vi "子VI-查看某框-只读穿透图模式.vi"(0 "输入框号（默认值0为整张图）":dbl format="%#_13g", 1 "框组":T3(array[cluster]), 2 "临界Z值":i32, 4 "临界面积百分比值":dbl, 5 "预先配置的灰度阈值":dbl, 6 "穿透图原始路径":path, 7 "部位信息":string[](array[string])=["", "34.500000", "32.500000", "1121", "34", "54.955926", "分层类", "不合格", ""], 12 "产品规格":cluster{"产品长度（周长）（mm）":dbl, "产品宽度（母线长）（mm）":dbl}) -> (14 "弥散类检测结果":string[][](table), 19 "分层类检测结果":string[][](table))   [LabVIEW 2021]
uses:
  <vilib>/vision/NI_Vision_Development_Module.lvlib
panel:
  in  "返回主界面":bool caption="辅助定性分析"
  out "Pixel Measurements":i32[](array[ring])=[0, 1, 2, 23, 24, 0, 1, 48] items=["Bounding Rect Width", "Bounding Rect Height", "Area"]
  in  "Tab Control":T1
  out "?":T2(plugin-control)
  out "Threshold Image":T2(plugin-control)
  out "Threshold Image":T2(plugin-control)
  in  "格式字符串 3":string="%f"
  in  "分隔符（'\\'代码显示） 2":string="\t"
  out "弥散和分层临界灰度值":i64
  out "弥散缺陷个数":i32
  out "分层缺陷个数":i32
  out "合格？ 弥散类":string="fencengThreshold"
  out "合格？分层类":string="fencengThreshold"
  out "弥散测量结果":dbl[][](array[numeric]) format="%.2f"
  out "?":string
  out "面积 (pixels)":i32
  in  "格式字符串 2":string="%f"
  in  "分隔符（'\\'代码显示）":string="\t"
  out "分层测量结果":dbl[][](array[numeric]) format="%.2f"
  out "缺陷初步分类的临界值":sgl format="%#.3f"
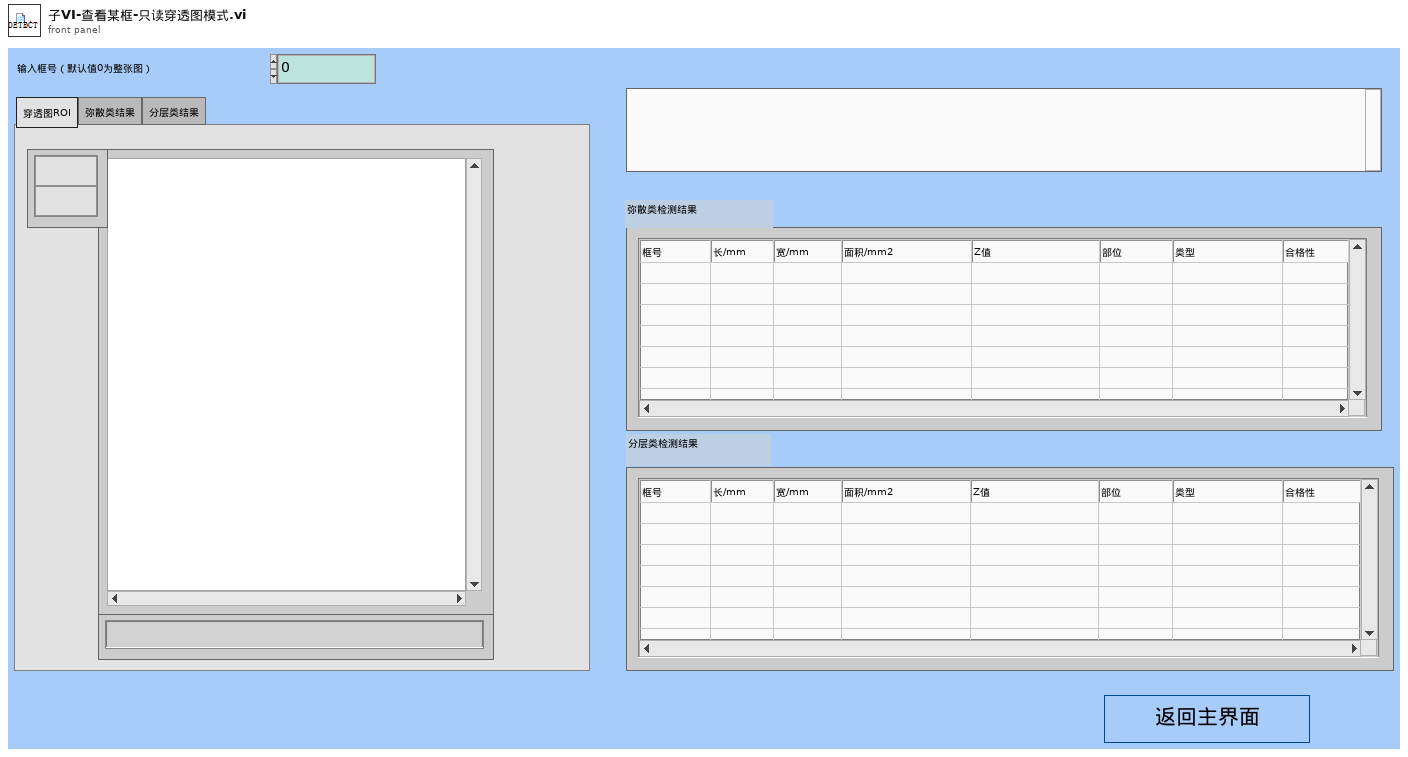
[diagram p1: front panel]
types:
  T1 = typedef "控件2.ctl" = enum32{"穿透图ROI", "弥散类结果", "分层类结果"}
  T2 = typedef "IMAQ Image.ctl" = refnum<image>
  T3 = cluster{"Global Rectangle":i32[], "Contours":cluster{"Contour Type":u32, "ROI Type":u32, "Points":i32[]}[]}[]
  T4 = cluster{"Zoom Tool":bool, "Selection Tool":bool, "Pan Tool":bool, "Point Tool":bool, "Line Tool":bool, "Rectangle Tool":bool, "Rotated Rectangle Tool":bool, "Polyline Tool":bool, "Polygon Tool":bool, "Freehand Tool":bool, "Closed Freehand Tool":bool, "Ellipse Tool":bool, "Annulus Tool":bool}
  T5 = typedef "Image Type" = u32
  T6 = cluster{"Global Rectangle":i32[], "Contours":cluster{"Contour Type":u32, "ROI Type":u32, "Points":i32[]}[]}
  T7 = typedef "Particle Parameters" = i32
  T8 = cluster{"Measurement Parameter":T7, "Range Lower Value":dbl, "Range Upper Value":dbl, "Range":bool, "Measurement Type":bool}[]
  T9 = cluster{"histogram":u32[], "Minimal Value":sgl, "Maximal Value":sgl, "Starting Value":sgl, "Interval Width":sgl, "Mean Value":sgl, "Standard  Variation":sgl, "Area (pixels)":i32}
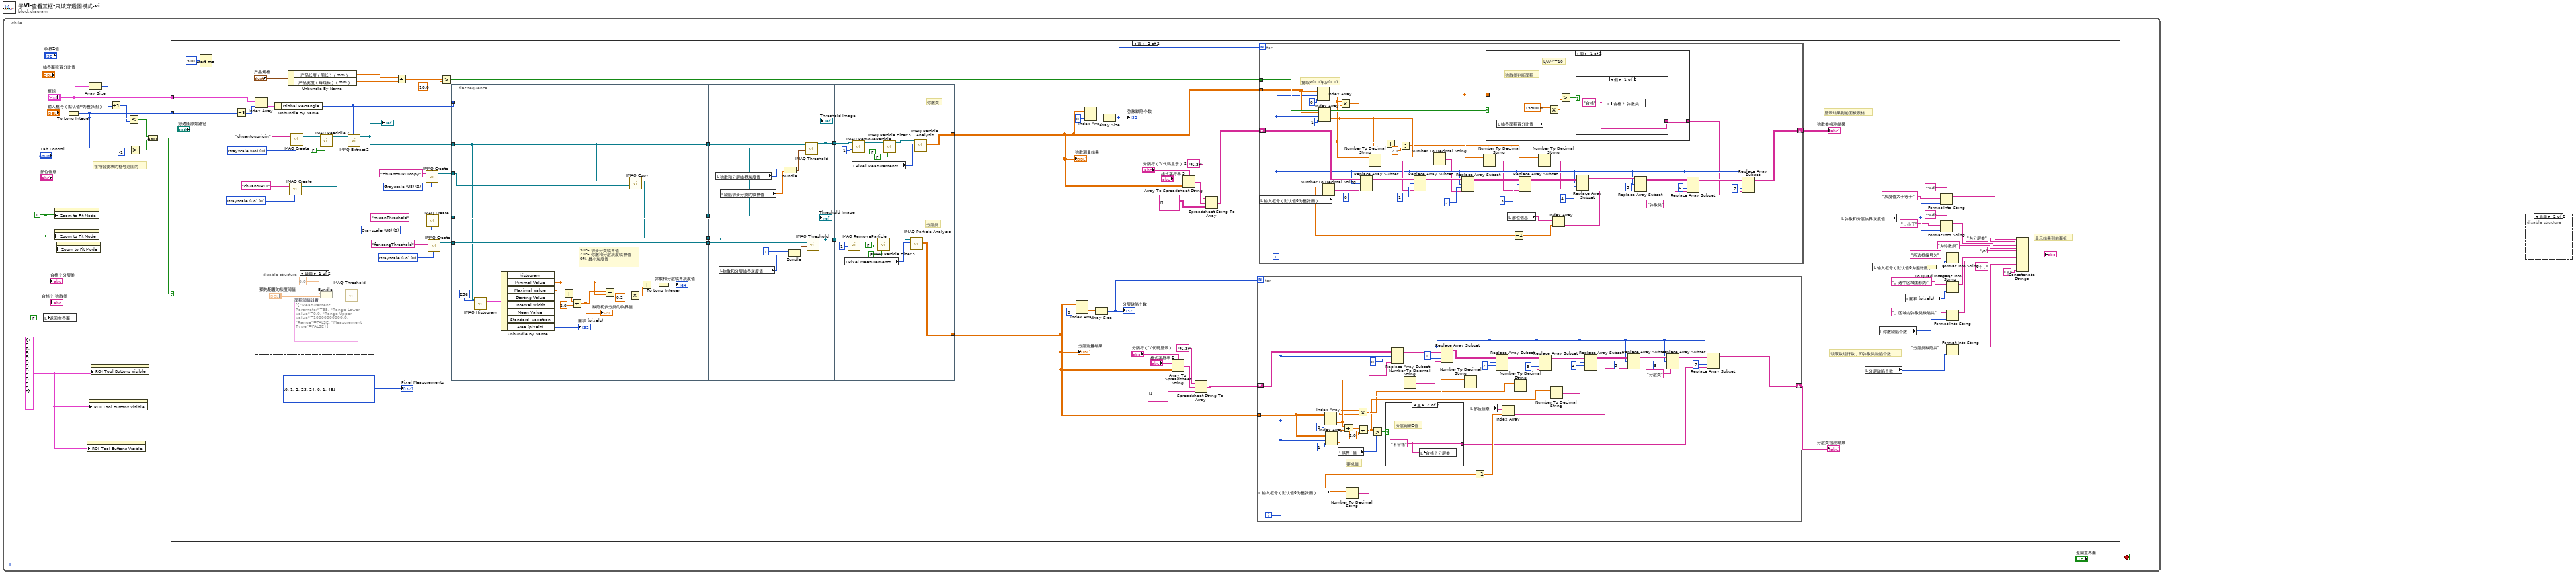
[diagram p0: block diagram]
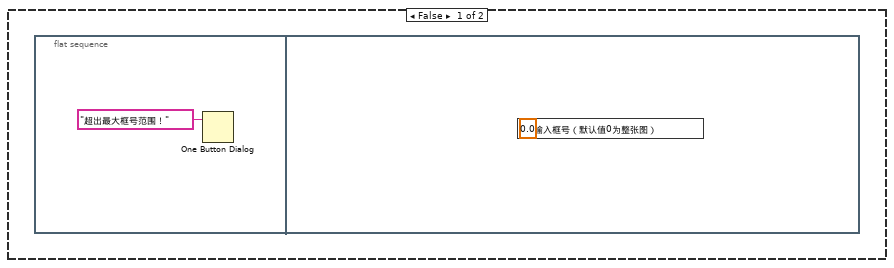
[diagram p2: hidden frame]
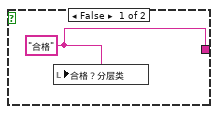
[diagram p4: hidden frame]
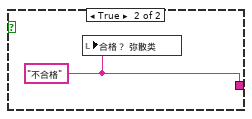
[diagram p5: hidden frame]
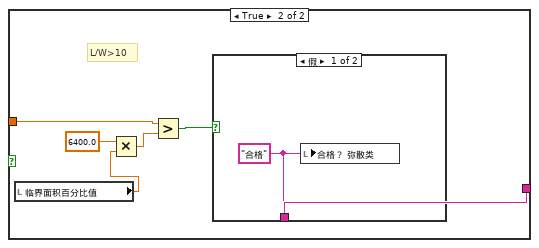
[diagram p6: hidden frame]
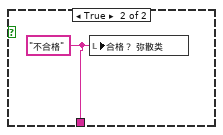
[diagram p7: hidden frame]
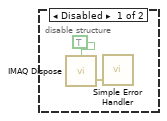
[diagram p8: hidden frame]
diagram:
  n1 = while {
    stop <- "返回主界面" stop-if-true
    w3 = T4 {"Zoom Tool"=TRUE, "Selection Tool"=FALSE, "Pan Tool"=TRUE, "Point Tool"=FALSE, "Line Tool"=FALSE, "Rectangle Tool"=FALSE, "Rotated Rectangle Tool"=FALSE, "Polyline Tool"=FALSE, "Polygon Tool"=FALSE, "Freehand Tool"=FALSE, "Closed Freehand Tool"=FALSE, "Ellipse Tool"=FALSE, "Annulus Tool"=FALSE} ("ROI Tool Buttons Visible:All Elements")
    w11 = TRUE ("Zoom to Fit Mode")
    # "在符合要求的框号范围内"
    n2 = local write "返回主界面"(FALSE ("stop")) -> ()
    n3 = property class="ImageControl"("Zoom to Fit Mode"=w11) -> ()  [unwired: 2 in, 2 out]
    n4 = property class="ImageControl"("Zoom to Fit Mode"=w11) -> ()  [unwired: 2 in, 2 out]
    n5 = property class="ImageControl"("Zoom to Fit Mode"=w11) -> ()  [unwired: 2 in, 2 out]
    n6 = To Long Integer(number="输入框号（默认值0为整张图）") -> (32bit integer=w5:i32)
    n7 = property class="ImageControl"("ROI Tool Buttons Visible"=w3) -> ()  [unwired: 2 in, 2 out]
    n8 = Array Size(array="框组") -> (size(s)=w2:i32)
    n9 = property class="ImageControl"("ROI Tool Buttons Visible"=w3) -> ()  [unwired: 2 in, 2 out]
    n10 = property class="ImageControl"("ROI Tool Buttons Visible"=w3) -> ()  [unwired: 2 in, 2 out]
    n11 = Increment(x=w2) -> (x+1=w1:i32)
    n12 = Less?(x=w5, y=w1) -> (x < y?=w7:bool)
    n13 = Greater?(x=w5, y=-1) -> (0:w6:bool)
    n14 = And(x=w7, y=w6) -> (x .and. y?=w8:bool)
    n15 = case shown="真" w8 {
      tunnel: "框组" -> [_ w18]
      tunnel: w5 -> [_ w17]
      frame False {
        n16 = flat-sequence {
          frame #0 {
            n17 = One Button Dialog(message="超出最大框号范围！" ("消息")) -> ()  [unwired: 1 in, 1 out]
          }
          frame #1 {
            n18 = local write "输入框号（默认值0为整张图）"(0.0 ("框号")) -> ()
          }
        }
      }
      frame True {
        w45 = T5 0 items=["Grayscale (U8)", "Grayscale (I16)", "Grayscale (SGL)", "Complex (CSG)", "RGB (U32)", "HSL (U32)", "RGB (U64)", "Grayscale (U16)"] ("Image Type")
        w74 = T5 0 items=["Grayscale (U8)", "Grayscale (I16)", "Grayscale (SGL)", "Complex (CSG)", "RGB (U32)", "HSL (U32)", "RGB (U64)", "Grayscale (U16)"] ("Image Type")
        w75 = T5 0 items=["Grayscale (U8)", "Grayscale (I16)", "Grayscale (SGL)", "Complex (CSG)", "RGB (U32)", "HSL (U32)", "RGB (U64)", "Grayscale (U16)"] ("Image Type")
        w78 = T5 0 items=["Grayscale (U8)", "Grayscale (I16)", "Grayscale (SGL)", "Complex (CSG)", "RGB (U32)", "HSL (U32)", "RGB (U64)", "Grayscale (U16)"] ("Image Type")
        w66 = i32[] [0, 1, 2, 23, 24, 0, 1, 48] items=["Bounding Rect Width", "Bounding Rect Height", "Area"] ("Pixel Measurements")
        w92 = T5 0 items=["Grayscale (U8)", "Grayscale (I16)", "Grayscale (SGL)", "Complex (CSG)", "RGB (U32)", "HSL (U32)", "RGB (U64)", "Grayscale (U16)"] ("Image Type")
        # "显示结果到前面板"
        # "读取数组行数，即弥散类缺陷个数"
        # "显示结果到前面板表格"
        n19 = Wait (ms)(milliseconds to wait=u32 500 ("等待时间（毫秒）")) -> ()  [unwired: 1 out]
        n20 = Decrement(x=w17) -> (x-1=w94:i32)
        n21 = Index Array(array=w18, index=w94) -> (element=w95:T6)
        n22 = disable-structure shown="禁用" {
          frame Disabled {
            (unwired) T8 [{"Measurement Parameter"=35, "Range Lower Value"=0.0, "Range Upper Value"=10000000000.0, "Range"=FALSE, "Measurement Type"=FALSE}]  # 面积阈值设置
            n23 = Bundle(0.0, "预先配置的灰度阈值"="预先配置的灰度阈值") -> ()  [unwired: 1 in, 1 out]
            n24 = call "IMAQ Threshold"() -> ()  [unwired: 6 in, 6 out]
          }
          frame Enabled {
          }
        }
        n25 = Unbundle By Name(w95) -> ("Global Rectangle"=w69:i32[])
        n26 = Unbundle By Name("产品规格") -> ("产品长度（周长）（mm）"=w86:dbl, "产品宽度（母线长）（mm）"=w85:dbl)
        n27 = call "IMAQ Create"("Image Name"="chuantuROI", "Image Type"=w78) -> ("New Image"=w77:T2)  [unwired: 3 in, 1 out]
        n28 = call "IMAQ Create"("Image Name"="chuantouorigin", "Image Type"=w92) -> ("New Image"=w80:T2)  [unwired: 3 in, 1 out]
        n29 = call "IMAQ ReadFile 2"("Use File Path Image Type"=FALSE, "File Path"="穿透图原始路径", "Image"=w80) -> ("Image Out"=w81:T2)  [unwired: 4 in, 4 out]
        n30 = call "IMAQ Extract 2"("Optional Rectangle"=w69, "Image Dst"=w77, "Image Src"=w81) -> ("Image Dst Out"=w48:T2)  [unwired: 7 in, 1 out]
        "?" <- w48
        n31 = Divide(x=w86, y=w85) -> (x/y=w89:dbl)
        n32 = call "IMAQ Create"("Image Name"="chuantouROIcopy", "Image Type"=w45) -> ("New Image"=w47:T2)  [unwired: 3 in, 1 out]
        n33 = call "IMAQ Create"("Image Name"="misanThreshold", "Image Type"=w74) -> ("New Image"=w68:T2)  [unwired: 3 in, 1 out]
        n34 = call "IMAQ Create"("Image Name"="fencengThreshold", "Image Type"=w75) -> ("New Image"=w67:T2)  [unwired: 3 in, 1 out]
        n35 = Greater?(x=w89, y=10.0) -> (0:w84:bool)
        n36 = flat-sequence {
          tunnel: [w163] -> w101
          tunnel: [w162] -> w100
          tunnel: [w148] -> w99
          tunnel: [w147] -> w98
          tunnel: w69 -> [_]
          tunnel: w68 -> [w163]
          tunnel: w67 -> [w162]
          tunnel: w48 -> [w148]
          tunnel: w47 -> [w146]
          tunnel: w101 -> [w175]
          tunnel: w100 -> [w174]
          tunnel: [w166] -> w97
          tunnel: [w167] -> w96
          tunnel: w99 -> [w168]
          tunnel: w98 -> [w165]
          tunnel: [w178] -> w51
          tunnel: [w189] -> w59
          tunnel: w97 -> [w184]
          tunnel: w96 -> [w181]
          frame #0 {
            # "50% 初步分类临界值\n20% 弥散和分层灰度临界值\n0% 最小灰度值"
            n37 = call "IMAQ Histogram"("Number of Classes"=256, "Image"=w148) -> ("Histogram Report"=w160:T9)  [unwired: 8 in, 1 out]
            n38 = Unbundle By Name(w160) -> ("Minimal Value"=w150:sgl, "Maximal Value"=w156:sgl, "Area (pixels)"=→"面积 (pixels)":i32)  [unwired: 5 out]
            n39 = Add(x=w150, y=w156) -> (x+y=w155:sgl)
            n40 = Divide(x=w155, y=sgl 2.0) -> (x/y=w154:sgl)
            "缺陷初步分类的临界值" <- w154
            n41 = Subtract(x=w154, y=w150) -> (x-y=w152:sgl)
            n42 = Multiply(x=w152, y=0.2) -> (x*y=w151:dbl)
            n43 = call "IMAQ Copy"("Image Dst"=w146, "Image Src"=w148) -> ("Image Dst Out"=w147:T2)  [unwired: 4 in, 1 out]
            n44 = Add(x=w150, y=w151) -> (x+y=w149:dbl)
            n45 = To Long Integer(number=w149) -> (32bit integer=→"弥散和分层临界灰度值":i32)
          }
          frame #1 {
            n46 = local read "弥散和分层临界灰度值"() -> (w164:i64)
            n47 = local read "弥散和分层临界灰度值"() -> (w170:i64)
            n48 = local read "缺陷初步分类的临界值"() -> (w172:sgl)
            n49 = Bundle("弥散和分层临界灰度值"=w164, "缺陷初步分类的临界值"=w172) -> (w173:cluster{"弥散和分层临界灰度值":i64, "缺陷初步分类的临界值":sgl})  [unwired: 1 in]
            n50 = Bundle(1, "弥散和分层临界灰度值"=w170) -> (w169:cluster{i32, "弥散和分层临界灰度值":i64})  [unwired: 1 in]
            n51 = call "IMAQ Threshold"("Range"=w173, "Image Dst"=w175, "Image Src"=w168) -> ("Image Dst Out"=w167:T2)  [unwired: 3 in, 5 out]
            "Threshold Image" <- w167
            n52 = call "IMAQ Threshold"("Range"=w169, "Image Dst"=w174, "Image Src"=w165) -> ("Image Dst Out"=w166:T2)  [unwired: 3 in, 5 out]
            "Threshold Image" <- w166
          }
          frame #2 {
            # "分层类"
            # "弥散类"
            n53 = local read "Pixel Measurements"() -> (w186:i32[])
            n54 = call "IMAQ RemoveParticle"("Number of Erosion"=1, "Image Src"=w184) -> ("Image Dst Out"=w185:T2)  [unwired: 8 in, 1 out]
            n55 = local read "Pixel Measurements"() -> (w187:i32[])
            n56 = call "IMAQ RemoveParticle"("Number of Erosion"=1, "Image Src"=w181) -> ("Image Dst Out"=w182:T2)  [unwired: 8 in, 1 out]
            n57 = call "IMAQ Particle Filter 3"("Image Src"=w185, "Keep/Remove Particles (F)"=FALSE, "Reject Border? (F)"=FALSE) -> ("Image Dst Out"=w188:T2)  [unwired: 10 in, 2 out]
            n58 = call "IMAQ Particle Filter 3"("Image Src"=w182, "Keep/Remove Particles (F)"=FALSE, "Reject Border? (F)"=FALSE) -> ("Image Dst Out"=w179:T2)  [unwired: 10 in, 2 out]
            n59 = call "IMAQ Particle Analysis"("Pixel Measurements"=w186, "Image"=w188) -> ("Particle Measurements (Pixels)"=w189:dbl[][])  [unwired: 4 in, 5 out]
            n60 = call "IMAQ Particle Analysis"("Pixel Measurements"=w187, "Image"=w179) -> ("Particle Measurements (Pixels)"=w178:dbl[][])  [unwired: 4 in, 5 out]
          }
        }
        n61 = Index Array(array=w59, index (col)=0 ("禁用的索引 (列)")) -> (element=w73:dbl[])  [unwired: 1 in]
        n62 = Index Array(array=w51, index (col)=0 ("禁用的索引 (列)")) -> (element=w71:dbl[])  [unwired: 1 in]
        n63 = Array Size(array=w73) -> (size(s)=w65:i32)
        "分层缺陷个数" <- w65
        n64 = Array Size(array=w71) -> (size(s)=w83:i32)
        "弥散缺陷个数" <- w83
        n65 = Array To Spreadsheet String(delimiter (Tab)="分隔符（'\\'代码显示）", array=w59, 3:"格式字符串 2") -> (spreadsheet string=w62:string)
        n66 = Array To Spreadsheet String(delimiter (Tab)="分隔符（'\\'代码显示） 2", array=w51, 3:"格式字符串 3") -> (spreadsheet string=w54:string)
        n67 = Spreadsheet String To Array(format string="%.3f", spreadsheet string=w62, array type (2D Dbl)=string[][] [] ("Array")) -> (array=w58:string[][])  [unwired: 1 in]
        n68 = Spreadsheet String To Array(format string="%.3f", spreadsheet string=w54, array type (2D Dbl)=string[][] [] ("Array")) -> (array=w50:string[][])  [unwired: 1 in]
        n69 = for {
          N: w65 -> [_]
          tunnel: w59 -> [w135]
          shift-right: [w113] -> w57
          shift-left: w58 -> [w124]
          i -> [w108]
          # "要求值"
          n70 = local read "输入框号（默认值0为整张图）"() -> (w133:dbl)
          n71 = Index Array(array=w135, index (row)=w108, index (col)=0 ("禁用的索引 (列)")) -> (element=w112:dbl)
          n72 = Index Array(array=w135, index (row)=w108, index (col)=1 ("禁用的索引 (列)")) -> (element=w111:dbl)
          n73 = local read "临界Z值"() -> (w141:i32)
          n74 = Add(x=w112, y=w111) -> (x+y=w142:dbl)
          n75 = Number To Decimal String(number=w133) -> (decimal integer string=w125:string)  [unwired: 1 in]
          n76 = Multiply(x=w112, y=w111) -> (x*y=w110:dbl)
          n77 = Divide(x=w142, y=2.0) -> (x/y=w107:dbl)
          n78 = Greater?(x=w107, y=w141) -> (0:w143:bool)
          n79 = case shown="真" w143 {
            tunnel: [w144 w145] -> w104
            frame False {
              w144 = "合格" ("合格？")
              n80 = local write "合格？分层类"(w144) -> ()
            }
            frame True {
              w145 = "不合格" ("合格？")
              # "分层判断Z值"
              n81 = local write "合格？分层类"(w145) -> ()
            }
          }
          n82 = Replace Array Subset(array=w124, new element=w125, index (row)=w108, index (col)=0 ("索引 (列)")) -> (w123:string[][])
          n83 = Number To Decimal String(number=w112) -> (decimal integer string=w122:string)  [unwired: 1 in]
          n84 = Replace Array Subset(array=w123, new element=w122, index (row)=w108, index (col)=1 ("索引 (列)")) -> (w120:string[][])
          n85 = Number To Decimal String(number=w111) -> (decimal integer string=w121:string)  [unwired: 1 in]
          n86 = local read "部位信息"() -> (w137:string[])
          n87 = Decrement(x=w133) -> (x-1=w136:dbl)
          n88 = Replace Array Subset(array=w120, new element=w121, index (row)=w108, index (col)=2 ("索引 (列)")) -> (w119:string[][])
          n89 = Index Array(array=w137, index=w136) -> (element=w106:string)
          n90 = Number To Decimal String(number=w110) -> (decimal integer string=w118:string)  [unwired: 1 in]
          n91 = Replace Array Subset(array=w119, new element=w118, index (row)=w108, index (col)=3 ("索引 (列)")) -> (w117:string[][])
          n92 = Number To Decimal String(number=w107) -> (decimal integer string=w109:string)  [unwired: 1 in]
          n93 = Replace Array Subset(array=w117, new element=w109, index (row)=w108, index (col)=4 ("索引 (列)")) -> (w116:string[][])
          n94 = Replace Array Subset(array=w116, new element=w106, index (row)=w108, index (col)=5 ("索引 (列)")) -> (w115:string[][])
          n95 = Replace Array Subset(array=w115, new element="分层类" ("新元素/子数组"), index (row)=w108, index (col)=6 ("索引 (列)")) -> (w114:string[][])
          n96 = Replace Array Subset(array=w114, new element=w104, index (row)=w108, index (col)=7 ("索引 (列)")) -> (w113:string[][])
        }
        "分层类检测结果" <- w57
        n97 = for {
          N: w83 -> [_]
          tunnel: w84 -> [w230]
          tunnel: w51 -> [w229]
          shift-right: [w209] -> w49
          shift-left: w50 -> [w217]
          i -> [w207]
          # "提取x(0,0)和y(0,1)"
          n98 = local read "输入框号（默认值0为整张图）"() -> (w195:dbl)
          n99 = Index Array(array=w229, index (row)=w207, index (col)=0 ("禁用的索引 (列)")) -> (element=w201:dbl)
          n100 = Index Array(array=w229, index (row)=w207, index (col)=1 ("禁用的索引 (列)")) -> (element=w200:dbl)
          n101 = Number To Decimal String(number=w195) -> (decimal integer string=w218:string)  [unwired: 1 in]
          n102 = Multiply(x=w201, y=w200) -> (x*y=w205:dbl)
          n103 = Replace Array Subset(array=w217, new element=w218, index (row)=w207, index (col)=0 ("索引 (列)")) -> (w216:string[][])
          n104 = Number To Decimal String(number=w201) -> (decimal integer string=w208:string)  [unwired: 1 in]
          n105 = Add(x=w201, y=w200) -> (x+y=w203:dbl)
          n106 = Divide(x=w203, y=2.0) -> (x/y=w199:dbl)
          n107 = Replace Array Subset(array=w216, new element=w208, index (row)=w207, index (col)=1 ("索引 (列)")) -> (w215:string[][])
          n108 = Number To Decimal String(number=w200) -> (decimal integer string=w206:string)  [unwired: 1 in]
          n109 = Replace Array Subset(array=w215, new element=w206, index (row)=w207, index (col)=2 ("索引 (列)")) -> (w214:string[][])
          n110 = Number To Decimal String(number=w205) -> (decimal integer string=w204:string)  [unwired: 1 in]
          n111 = case shown="假" w230 {
            tunnel: w205 -> [w236 w244]
            tunnel: [w234 w242] -> w192
            frame False {
              # "弥散类判断面积"
              # "L/W<=10"
              n112 = local read "临界面积百分比值"() -> (w232:dbl)
              n113 = Multiply(x=15500.0, y=w232) -> (x*y=w231:dbl)
              n114 = Greater?(x=w236, y=w231) -> (0:w235:bool)
              n115 = case shown="假" w235 {
                tunnel: [w237 w238] -> w234
                frame False {
                  w237 = "合格" ("合格？")
                  n116 = local write "合格？ 弥散类"(w237) -> ()
                }
                frame True {
                  w238 = "不合格" ("合格？")
                  n117 = local write "合格？ 弥散类"(w238) -> ()
                }
              }
            }
            frame True {
              # "L/W>10"
              n118 = local read "临界面积百分比值"() -> (w239:dbl)
              n119 = Multiply(x=6400.0, y=w239) -> (x*y=w241:dbl)
              n120 = Greater?(x=w244, y=w241) -> (0:w243:bool)
              n121 = case shown="假" w243 {
                tunnel: [w245 w246] -> w242
                frame False {
                  w245 = "合格" ("合格？")
                  n122 = local write "合格？ 弥散类"(w245) -> ()
                }
                frame True {
                  w246 = "不合格" ("合格？")
                  n123 = local write "合格？ 弥散类"(w246) -> ()
                }
              }
            }
          }
          n124 = local read "部位信息"() -> (w197:string[])
          n125 = Decrement(x=w195) -> (x-1=w196:dbl)
          n126 = Replace Array Subset(array=w214, new element=w204, index (row)=w207, index (col)=3 ("索引 (列)")) -> (w213:string[][])
          n127 = Number To Decimal String(number=w199) -> (decimal integer string=w198:string)  [unwired: 1 in]
          n128 = Index Array(array=w197, index=w196) -> (element=w194:string)
          n129 = Replace Array Subset(array=w213, new element=w198, index (row)=w207, index (col)=4 ("索引 (列)")) -> (w212:string[][])
          n130 = Replace Array Subset(array=w212, new element=w194, index (row)=w207, index (col)=5 ("索引 (列)")) -> (w211:string[][])
          n131 = Replace Array Subset(array=w211, new element="弥散类" ("新元素/子数组"), index (row)=w207, index (col)=6 ("索引 (列)")) -> (w210:string[][])
          n132 = Replace Array Subset(array=w210, new element=w192, index (row)=w207, index (col)=7 ("索引 (列)")) -> (w209:string[][])
        }
        "弥散类检测结果" <- w49
        n133 = local read "弥散和分层临界灰度值"() -> (w44:i64)
        n134 = local read "分层缺陷个数"() -> (w20:i32)
        n135 = local read "输入框号（默认值0为整张图）"() -> (w35:dbl)
        n136 = local read "弥散缺陷个数"() -> (w19:i32)
        n137 = local read "面积 (pixels)"() -> (w38:i32)
        n138 = To Quad Integer(1:w35) -> (0:w36:i64)
        n139 = Format Into String(format string="%d" ("格式字符串"), initial string="灰度值大于等于" ("初始字符串"), w44) -> (resulting string=w40:string)  [unwired: 1 in, 1 out]
        n140 = Format Into String(format string="%d" ("格式字符串"), initial string="，小于" ("初始字符串"), w44) -> (resulting string=w39:string)  [unwired: 1 in, 1 out]
        n141 = Format Into String(initial string="所选框编号为" ("初始字符串"), w36) -> (resulting string=w34:string)  [unwired: 2 in, 1 out]
        n142 = Format Into String(initial string="。选中区域面积为" ("字符串"), w38) -> (resulting string=w41:string)  [unwired: 2 in, 1 out]
        n143 = Format Into String(initial string="。区域内弥散类缺陷共" ("初始字符串"), w19) -> (resulting string=w42:string)  [unwired: 2 in, 1 out]
        n144 = Format Into String(initial string="分层类缺陷共" ("初始字符串"), w20) -> (resulting string=w43:string)  [unwired: 2 in, 1 out]
        n145 = Concatenate Strings(w40, "为分层类" ("初始字符串"), w39, "为弥散类" ("初始字符串"), "\n", w34, w41, w42, "个，" ("字符串"), w43, "个" ("字符串")) -> (→"?":string)
        "分层测量结果" <- w59
        "弥散测量结果" <- w51
        "Pixel Measurements" <- w66
      }
    }
  }
  n146 = disable-structure shown="启用" {
    frame Disabled {
      n147 = call "IMAQ Dispose"("All Images? (No)"=TRUE) -> ("error out"=w248:errorcluster)  [unwired: 5 in]
      n148 = call <vilib>:"Simple Error Handler.vi"("error in (no error)"=w248) -> ()  [unwired: 4 in, 5 out]
    }
    frame Enabled {
    }
  }
